vi "Fix Lidar Values.vi"(11 "Distances In":dbl[](array[numeric])) -> (3 "Distances Out":dbl[](array[numeric]))   [LabVIEW 2011]
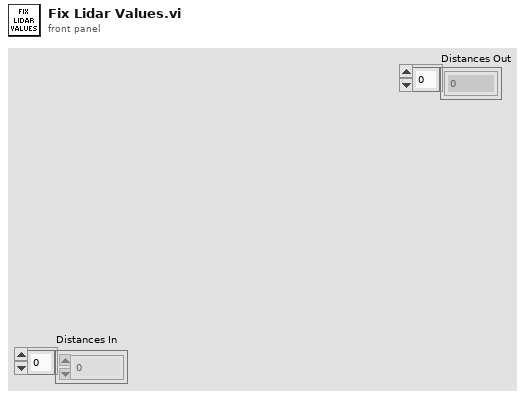
[diagram p1: front panel]
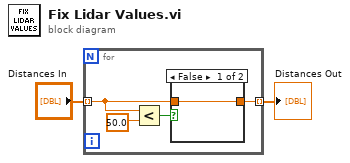
[diagram p0: block diagram]
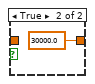
[diagram p2: hidden frame]
diagram:
  n1 = for {
    tunnel: "Distances In" -> [w4] mode=indexing
    tunnel: [w3] -> w1 mode=indexing
    n2 = Less?(x=w4, y=50.0) -> (x < y?=w5:bool)
    n3 = case shown="False" w5 {
      tunnel: w4 -> [w7 _]
      tunnel: [w7 30000.0] -> w3
      frame False {
      }
      frame True {
      }
    }
  }
  "Distances Out" <- w1
